vi "Aurora Writer (Dual Port).vi"(0 "input":bool[](array[boolean]), 2 "aurora tx dual reference":T1, 9 "input valid":bool) -> (14 "ready for input":bool)   [LabVIEW 2019]
uses:
  <vilib>/eio/EIONode/EIONode.xnode
  <instrlib>/_niInstr/Data Formatting/v1/FPGA/niInstr Data Formatting v1 FPGA.lvlib
  <instrlib>/_niInstr/Data Formatting/v1/FPGA/Private/Convert/Boolean Array to U64 Array.vi
  <vilib>/rvi/eio/common/nirviEmuTemplateMethod_errors.vi
  Aurora TX Dual Reference.ctl
  AXI4-Stream Writer FXP64x4 Resources.ctl
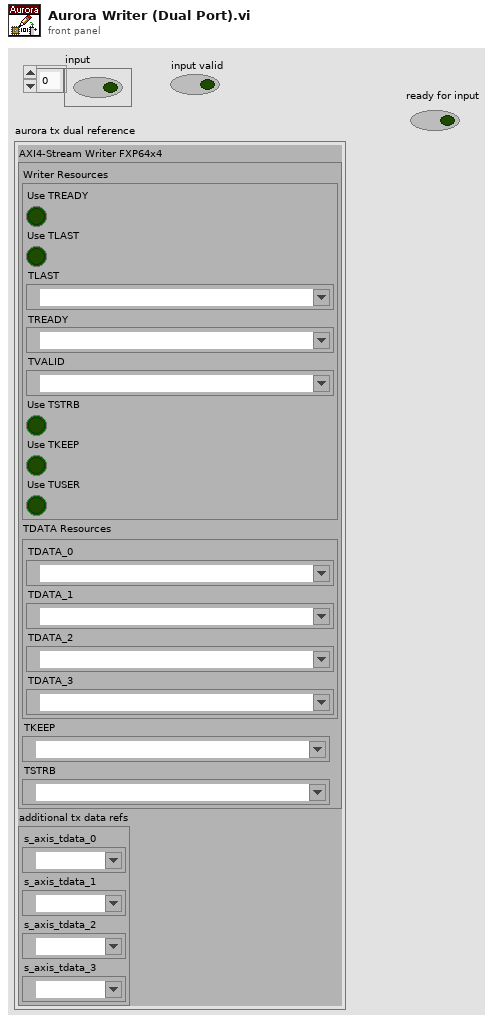
[diagram p1: front panel]
types:
  T1 = typedef "Aurora TX Dual Reference.ctl" = cluster{"AXI4-Stream Writer FXP64x4":T2, "additional tx data refs":cluster{"s_axis_tdata_0":refnum<k21>, "s_axis_tdata_1":refnum<k21>, "s_axis_tdata_2":refnum<k21>, "s_axis_tdata_3":refnum<k21>}}
  T2 = typedef "AXI4-Stream Writer FXP64x4 Resources.ctl" = cluster{"Writer Resources":cluster{"Use TREADY":bool, "Use TLAST":bool, "TLAST":refnum<k21>, "TREADY":refnum<k21>, "TVALID":refnum<k21>, "Use TSTRB":bool, "Use TKEEP":bool, "Use TUSER":bool}, "TDATA Resources":cluster{"TDATA_0":refnum<k21>, "TDATA_1":refnum<k21>, "TDATA_2":refnum<k21>, "TDATA_3":refnum<k21>}, "TKEEP":refnum<k21>, "TSTRB":refnum<k21>}
  T3 = cluster{"s_axis_tdata_0":refnum<k21>, "s_axis_tdata_1":refnum<k21>, "s_axis_tdata_2":refnum<k21>, "s_axis_tdata_3":refnum<k21>}
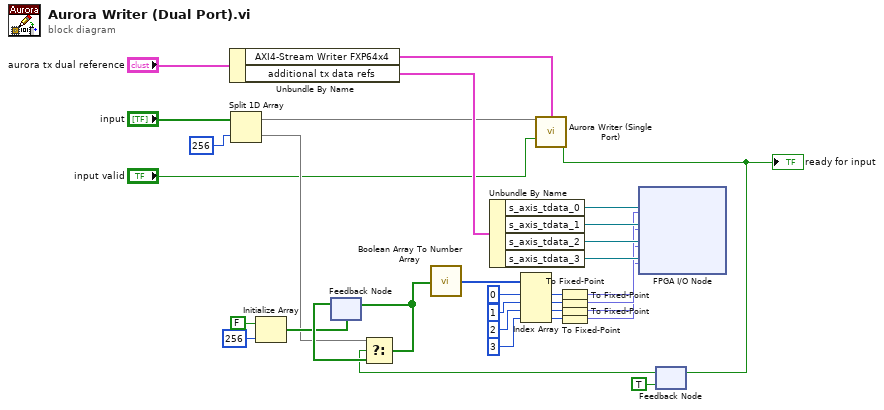
[diagram p0: block diagram]
diagram:
  n1 = Unbundle By Name("aurora tx dual reference") -> ("AXI4-Stream Writer FXP64x4"=w4:T2, "additional tx data refs"=w32:T3)
  n2 = Split 1D Array(array="input", index=256) -> (first subarray=w3:bool[], second subarray=w5:bool[])
  n3 = Initialize Array(FALSE ("TLAST Value"), 256 ("dimension size")) -> (w22:bool[])
  n4 = feedback #1(w22) -> (w24:bool[])
  n5 = Unbundle By Name(w32) -> ("s_axis_tdata_0"=w29:refnum<k21>, "s_axis_tdata_1"=w28:refnum<k21>, "s_axis_tdata_2"=w27:refnum<k21>, "s_axis_tdata_3"=w26:refnum<k21>)
  n6 = call "Aurora Writer (Single Port).vi"("input data"=w3, "AXI4-Stream Writer FXP64x4"=w4, "input valid"="input valid") -> ("ready for input"=w1:bool)  [unwired: 12 in]
  "ready for input" <- w1
  n7 = feedback #2(TRUE) -> (w21:bool)
  n8 = Select(t=w5, s=w21, f=w24) -> (s? t:f=w11:bool[])
  n9 = feedback-in #1(w11) -> ()
  n10 = call-poly <instrlib>:"Boolean Array To Number Array.vi"("data in"=w11) -> ("data out"=w16:u64[])  [unwired: 14 in]
  n11 = Index Array(array=w16, index #1=0 ("index"), index #2=1 ("index"), index #3=2 ("index"), index #4=3 ("index")) -> (element #1=w15:u64, element #2=w14:u64, element #3=w13:u64, element #4=w12:u64)
  n12 = To Fixed-Point(number=w15) -> (fixed-point=w10:fxp<+,64,64>)  [unwired: 1 in]
  n13 = To Fixed-Point(number=w14) -> (fixed-point=w9:fxp<+,64,64>)  [unwired: 1 in]
  n14 = To Fixed-Point(number=w13) -> (fixed-point=w8:fxp<+,64,64>)  [unwired: 1 in]
  n15 = To Fixed-Point(number=w12) -> (fixed-point=w7:fxp<+,64,64>)  [unwired: 1 in]
  n16 = xnode "FPGA I/O Node"("I/O Item"=w10, "FPGA I/O In"=w29, "I/O Item"=w9, "FPGA I/O In"=w28, "I/O Item"=w8, "FPGA I/O In"=w27, "I/O Item"=w7, "FPGA I/O In"=w26) -> ()  [unwired: 4 out]
  n17 = feedback-in #2(w1) -> ()
